vi "2D DCT.vi"(11 "X":dbl[][](array[numeric])) -> (0 "error":i32, 3 "DCT {X}":dbl[][](array[numeric]))   [LabVIEW 2010, in "NI_AALPro.lvlib"]
doc: "Computes the Discrete Cosine Transform (DCT) of the input sequence <B>X</B>. Wire data to the <B>X</B> input to determine the polymorphic instance to use or manually select the instance."
uses:
  NI_AALPro.lvlib
  lvanlys.dll
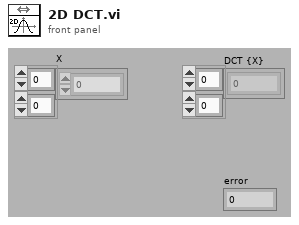
[diagram p1: front panel]
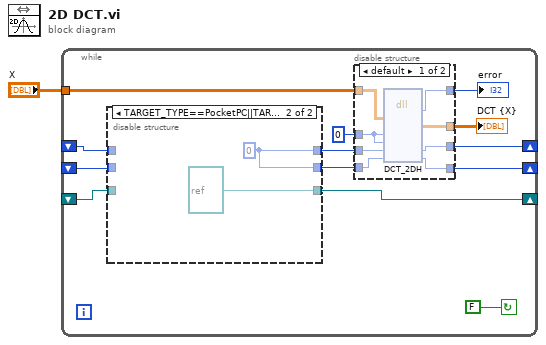
[diagram p0: block diagram]
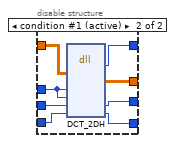
[diagram p2: hidden frame]
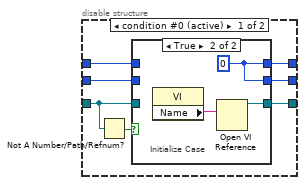
[diagram p3: hidden frame]
diagram:
  n1 = while {
    shift-left: _ -> [w13]
    shift-right: [w4] -> _
    tunnel: "X" -> [w3]
    shift-right: [w12] -> _
    shift-left: _ -> [w11]
    shift-right: [w5] -> _
    shift-left: _ -> [w8]
    stop <- FALSE continue-if-true
    n2 = disable-structure shown="TARGET_TYPE==PocketPC||TARGET_TYPE==PalmOS||TARGET_TYPE==FPGA||TARGET_TYPE==Embedded" {
      disable-tunnel: w11 -> [w35 _]
      disable-tunnel: [w36 refnum<vi> refnum ("VI Refnum")] -> w12
      disable-tunnel: w13 -> [w34 _]
      disable-tunnel: [w33 w45] -> w7
      disable-tunnel: w8 -> [w32 _]
      disable-tunnel: [w31 w45] -> w6
      frame condition #0 (active) {
        n3 = Not A Number/Path/Refnum?(number/path/refnum=w35) -> (NaN/Path/Refnum?=w37:bool)
        n4 = case shown="True" w37 {
          tunnel: [w40 w43] -> w36
          tunnel: w35 -> [w40 _]
          tunnel: w34 -> [w39 _]
          tunnel: [w39 w42] -> w33
          tunnel: w32 -> [w38 _]
          tunnel: [w38 w42] -> w31
          frame False {
          }
          frame True {
            w42 = 0 ("error")
            # "Initialize Case"
            n5 = property class="VI"() -> ("Name"=w41:string)  [unwired: 2 in, 2 out]
            n6 = Open VI Reference(vi path=w41) -> (vi reference=w43:refnum<vi>)  [unwired: 5 in, 1 out]
          }
        }
      }
      frame condition #1 {
        w45 = 0 ("t")
      }
    }
    n7 = disable-structure shown="default" {
      disable-tunnel: [w22 w30] -> w10
      disable-tunnel: [w21 w29] -> w9
      disable-tunnel: w7 -> [w20 w28]
      disable-tunnel: w6 -> [w19 w27]
      disable-tunnel: [w18 w26] -> w5
      disable-tunnel: [w17 w25] -> w4
      disable-tunnel: w3 -> [w16 w24]
      disable-tunnel: 0 ("m") -> [w15 w23]
      frame condition #0 {
        n8 = dll-call lib="C:/Program Files/National Instruments/LabVIEW 2010/resource/lvanlys.*" fn="DCT_2DH"("xH"=w16, "m"=w15, "n"=w15, "tbl1"=w20, "tbl2"=w19) -> (w22:i32, "yH"=w21:dbl[][], "tbl1"=w17:i32, "tbl2"=w18:i32)  [unwired: 7 in, 2 out]
      }
      frame condition #1 (active) {
        n9 = dll-call lib="C:/Program Files/National Instruments/LabVIEW 2010/resource/lvanlys.dll" fn="DCT_2DH"("xH"=w24, "m"=w23, "n"=w23, "tbl1"=w28, "tbl2"=w27) -> ("return type"=w30:i32, "yH"=w29:dbl[][], "tbl1"=w25:i64, "tbl2"=w26:i64)  [unwired: 7 in, 2 out]
      }
    }
    "error" <- w10
    "DCT {X}" <- w9
  }
